vi "DIAdem Open Connection.vi"(8 "error in (no error)":errorcluster) -> (0 "error out":errorcluster, 3 "DIAdem Reference":T1)   [LabVIEW 2020]
doc: "This VI opens a connection to a DIAdem application on the same computer. DIAdem must be installed. If DIAdem is not already running, it is opened by the VI."
uses:
  <vilib>/ExportToExcel/DIAdem Reference.ctl
panel:
  in  "milliseconds to wait":u32=200
  in  "DIAdem Reference":T1
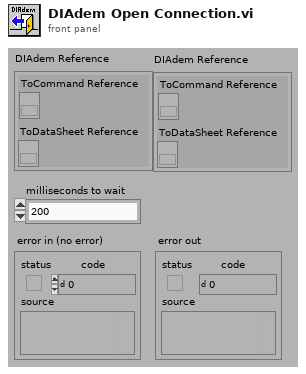
[diagram p1: front panel]
types:
  T1 = typedef "DIAdem Reference.ctl" = cluster{"ToCommand Reference":refnum<k7>, "ToDataSheet Reference":refnum<k7>}
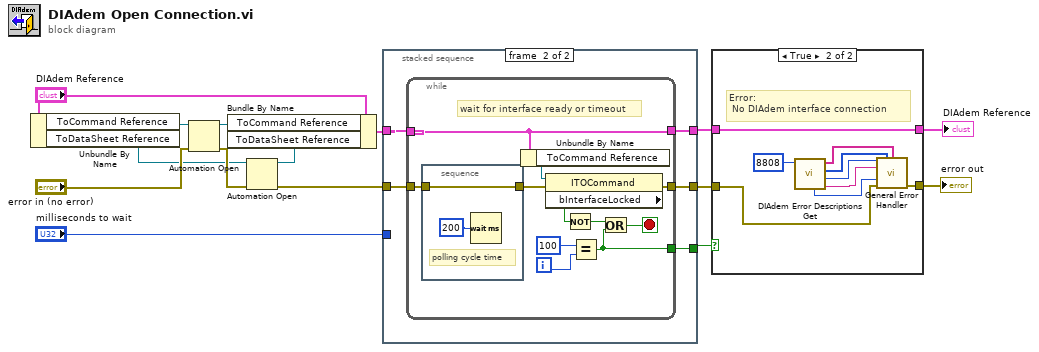
[diagram p0: block diagram]
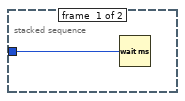
[diagram p2: hidden frame]
diagram:
  n1 = Unbundle By Name("DIAdem Reference") -> ("ToCommand Reference"=w12:refnum<k7>, "ToDataSheet Reference"=w11:refnum<k7>)
  n2 = Automation Open(error in (no error)="error in (no error)", Automation Refnum=w12) -> (Automation Refnum=w9:refnum<k7>, error out=w13:errorcluster)  [unwired: 2 in]
  n3 = Automation Open(error in (no error)=w13, Automation Refnum=w11) -> (Automation Refnum=w10:refnum<k7>, error out=w5:errorcluster)  [unwired: 2 in]
  n4 = Bundle By Name(cluster="DIAdem Reference", "ToCommand Reference"=w9, "ToDataSheet Reference"=w10) -> (w6:T1)
  n5 = stacked-sequence {
    tunnel: w6 -> [_ w21]
    tunnel: w5 -> [_ w20]
    tunnel: [_ w19] -> w4
    tunnel: [_ w18] -> w3
    tunnel: [_ w17] -> w2
    tunnel: "milliseconds to wait" -> [w16 _]
    frame #0 {
      n6 = Wait (ms)(milliseconds to wait=w16) -> ()  [unwired: 1 out]
    }
    frame #1 {
      n7 = while {
        tunnel: w21 -> [w24]
        tunnel: w20 -> [w23]
        tunnel: [w25] -> w17
        tunnel: [w27] -> w18
        tunnel: [w24] -> w19
        i -> [w30]
        stop <- w31 stop-if-true
        # "wait for interface ready or timeout"
        n8 = stacked-sequence {
          tunnel: w23 -> [w33]
          tunnel: [w33] -> w22
          frame #0 {
            # "polling cycle time"
            n9 = Wait (ms)(milliseconds to wait=u32 200) -> ()  [unwired: 1 out]
          }
        }
        n10 = Unbundle By Name(w24) -> ("ToCommand Reference"=w26:refnum<k7>)
        n11 = property class="ITOCommand"(reference=w26, error in=w22) -> (error out=w27:errorcluster, "bInterfaceLocked"=w28:bool)  [unwired: 1 out]
        n12 = Not(x=w28) -> (.not. x?=w32:bool)
        n13 = Equal?(x=100, y=w30) -> (x = y?=w25:bool)
        n14 = Or(x=w32, y=w25) -> (x .or. y?=w31:bool)
      }
    }
  }
  n15 = case shown="True" w2 {
    tunnel: w3 -> [w35 w44]
    tunnel: [w35 w43] -> w8
    tunnel: w4 -> [w36 w45]
    tunnel: [w36 w45] -> w7
    frame False {
    }
    frame True {
      # "Error:\n No DIAdem interface connection"
      n16 = call <vilib>:"DIAdem Error Descriptions Get.vi"("internal error code"=8808 ("[error code] (0)")) -> ("error source"=w39:string, "error code"=w40:i32, "DIAdem error codes"=w41:i32[], "DIAdem error descriptions"=w42:string[], "type of dialog"=w38:u16)  [unwired: 5 in, 1 out]
      n17 = call <vilib>:"General Error Handler.vi"("[error code] (0)"=w40, "[user-defined codes]"=w41, "[user-defined descriptions]"=w42, "[error source] (\" \")"=w39, "type of dialog (OK msg:1)"=w38, "error in (no error)"=w44) -> ("error out"=w43:errorcluster)  [unwired: 5 in, 4 out]
    }
  }
  "error out" <- w8
  "DIAdem Reference" <- w7
